vi "add gating initalize(SubVI).vi"(9 "字符串":string, 10 "model":string="Delta") -> (0 "连接的字符串":string, 3 "ok or cancel":bool=TRUE)   [LabVIEW 2019, in "Add Seq.lvlib"]
uses:
  Add Seq.lvlib
  SubVI.lvlib
panel:
  in  "Compliance  Level (A)":dbl=0.0001
  in  "2400 resource name":refnum<visa-resource-name>
  out "错误输出":errorcluster
  in  "load":bool
  in  "cancel":bool
  in  "ok":bool
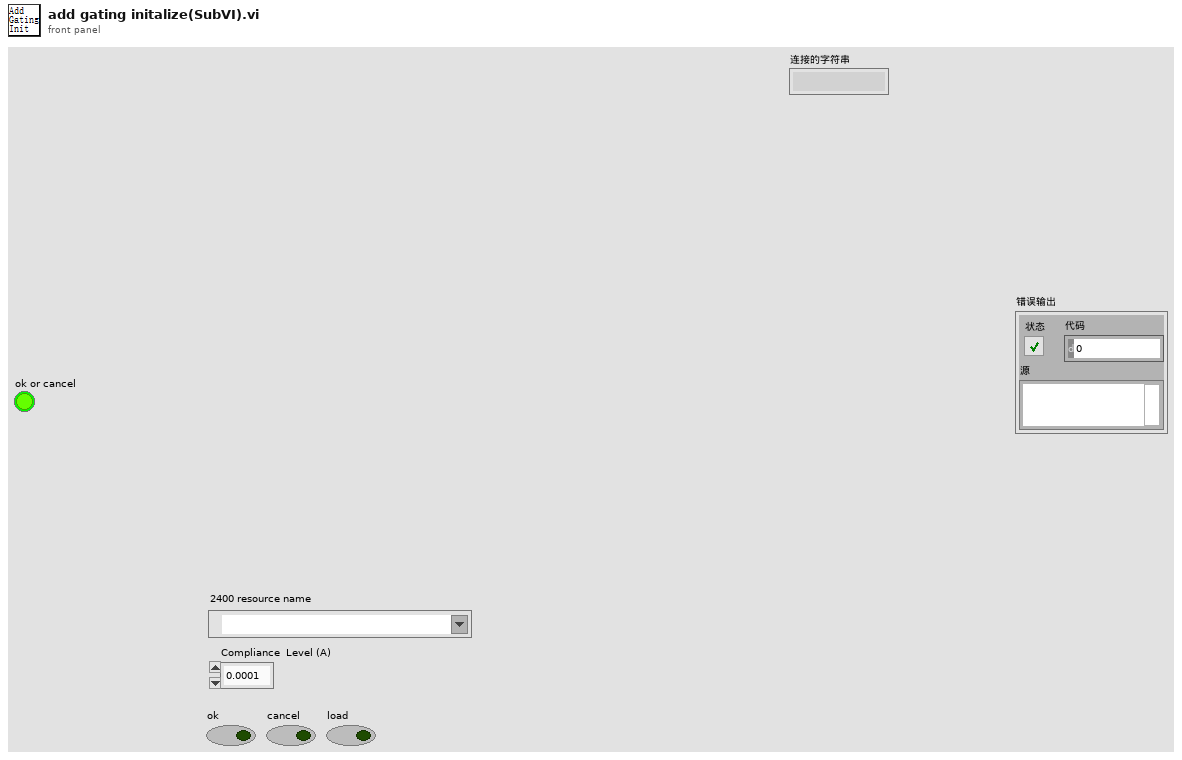
[diagram p1: front panel]
types:
  T1 = enum16{"open", "replace", "create", "open or create", "replace or create"}
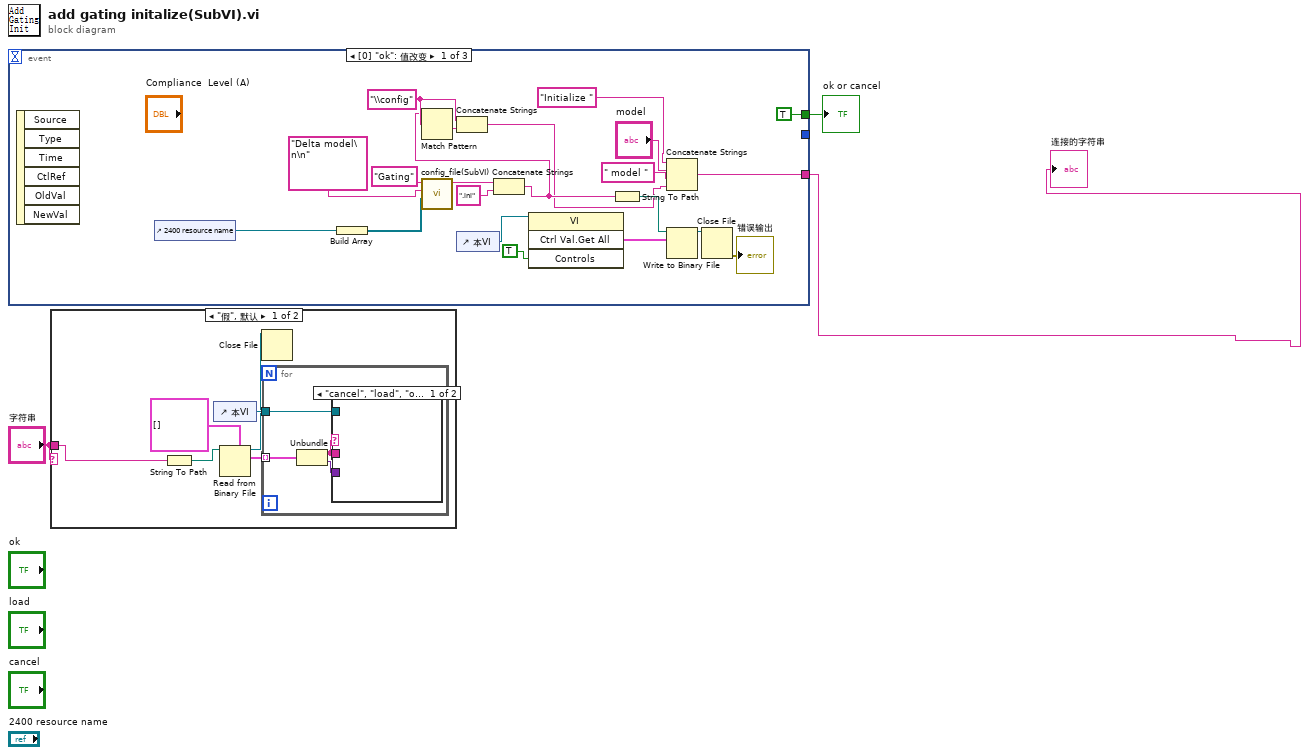
[diagram p0: block diagram]
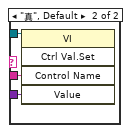
[diagram p2: hidden frame]
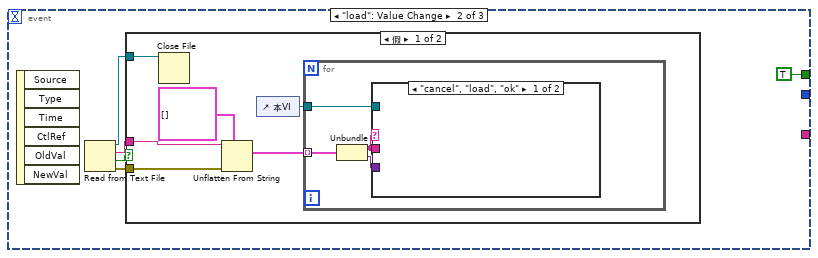
[diagram p4: hidden frame]
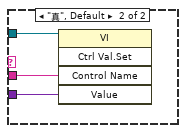
[diagram p5: hidden frame]
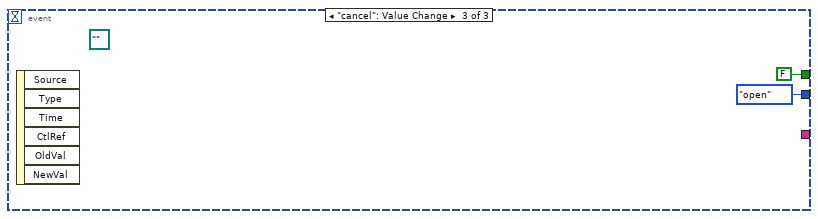
[diagram p7: hidden frame]
diagram:
  n1 = event shown="[0] \"ok\": 值改变" {
    selector: _ -> [_ _ _]
    dyn-events: _ -> [_ _ _]
    timeout: _ -> [_ _ _]
    tunnel: [_ _ T1."open" ("operation(0:open)")] -> _
    tunnel: [TRUE TRUE FALSE] -> w3
    tunnel: [w12 _ _] -> w1
    event "ok": Value Change {
      w7 = "\\config" ("正则表达式")
      n2 = event-data() -> ()  [unwired: 1 in, 6 out]
      n3 = control-ref of="2400 resource name"() -> (w8:refnum<vi>)
      n4 = Build Array(w8) -> (w15:refnum<vi>[])
      n5 = call "config_file(SubVI).vi"("all ref"=w15, "文件抬头"="Delta model\n\n", "文件夹名称"="Gating" ("字符串")) -> ("字符串输出"=w18:string)  [unwired: 8 in]
      n6 = control-ref of="本VI"() -> (w21:refnum<vi>)
      n7 = Concatenate Strings(w18, ".ini" ("字符串")) -> (w5:string)
      n8 = Match Pattern(string=w5, regular expression=w7) -> (after substring=w6:string)  [unwired: 1 in, 3 out]
      n9 = Concatenate Strings(w7, w6) -> (w4:string)
      n10 = invoke class="VI" method="Ctrl Val.Get All"(reference=w21, "Controls"=TRUE ("控件")) -> ("Get All Control Values Variant"=w10:cluster{"Name":string, "Variant Data":variant}[])  [unwired: 2 in, 3 out]
      n11 = String To Path(string=w5) -> (path=w11:path)
      n12 = Concatenate Strings("Initialize " ("字符串"), "model", " model " ("字符串"), w4) -> (w12:string)
      n13 = Write to Binary File(file (use dialog)=w11, data=w10) -> (refnum out=w9:refnum<file>)  [unwired: 4 in, 2 out]
      n14 = Close File(refnum=w9) -> (error out=→"错误输出":errorcluster)  [unwired: 1 in, 1 out]
    }
    event "load": Value Change {
      n15 = event-data() -> ()  [unwired: 1 in, 6 out]
      n16 = Read from Text File() -> (refnum out=w28:refnum<file>, text=w26:string, cancelled=w25:bool, error out=w27:errorcluster)  [unwired: 4 in]
      n17 = case shown="假" w25 {
        tunnel: w28 -> [w35 _]
        tunnel: w27 -> [w33 _]
        tunnel: w26 -> [w32 _]
        frame False {
          n18 = Close File(refnum=w35) -> ()  [unwired: 1 in, 2 out]
          n19 = Unflatten From String(type=cluster{"Name":string, "Variant Data":variant}[] [] ("控件值:获取全部"), binary string=w32, error in (no error)=w33) -> (value=w31:cluster{"Name":string, "Variant Data":variant}[])  [unwired: 2 in, 2 out]
          n20 = control-ref of="本VI"() -> (w30:refnum<vi>)
          n21 = for {
            tunnel: w31 -> [w39] mode=indexing
            tunnel: w30 -> [w38]
            n22 = Unbundle(w39) -> ("Name"=w36:string, "Variant Data"=w37:variant)
            n23 = case shown="\"cancel\", \"load\", \"ok\"" w36 {
              tunnel: w38 -> [_ w42]
              tunnel: w36 -> [_ w41]
              tunnel: w37 -> [_ w40]
              frame "cancel", "load", "ok" {
              }
              frame "真", Default {
                n24 = invoke class="VI" method="Ctrl Val.Set"(reference=w42, "Control Name"=w41, "Value"=w40) -> ()  [unwired: 2 in, 5 out]
              }
            }
          }
        }
        frame True {
        }
      }
    }
    event "cancel": Value Change {
      (unwired) path "" ("path")
      n25 = event-data() -> ()  [unwired: 1 in, 6 out]
    }
  }
  "ok or cancel" <- w3
  "连接的字符串" <- w1
  n26 = case shown="\"假\", 默认" "字符串" {
    tunnel: "字符串" -> [w50 _]
    frame "假", Default {
      n27 = String To Path(string=w50) -> (path=w48:path)
      n28 = control-ref of="本VI"() -> (w49:refnum<vi>)
      n29 = Read from Binary File(5:cluster{"Name":string, "Variant Data":variant}[] [] ("控件值:获取全部"), 11:w48) -> (2:w46:cluster{"Name":string, "Variant Data":variant}[], 3:w45:refnum<file>)  [unwired: 4 in, 2 out]
      n30 = Close File(refnum=w45) -> ()  [unwired: 1 in, 2 out]
      n31 = for {
        tunnel: w46 -> [w54] mode=indexing
        tunnel: w49 -> [w53]
        n32 = Unbundle(w54) -> ("Name"=w51:string, "Variant Data"=w52:variant)
        n33 = case shown="\"cancel\", \"load\", \"ok\"" w51 {
          tunnel: w53 -> [_ w57]
          tunnel: w51 -> [_ w56]
          tunnel: w52 -> [_ w55]
          frame "cancel", "load", "ok" {
          }
          frame "真", Default {
            n34 = invoke class="VI" method="Ctrl Val.Set"(reference=w57, "Control Name"=w56, "Value"=w55) -> ()  [unwired: 2 in, 5 out]
          }
        }
      }
    }
    frame "" {
    }
  }
